vi "Get unpacked Excel file data.vi"(8 "Error In":errorcluster, 10 "temp zip path":path, 11 "Unzipped files":path[](array[path])) -> (0 "Error Out":errorcluster, 1 "workbook.xml path":path, 2 "sheet file names":string[](array[string]), 3 "sheet paths":path[](array[path]), 7 "sharedStrings path":path)   [LabVIEW 2021, in "Files.lvlib"]
uses:
  Files.lvlib
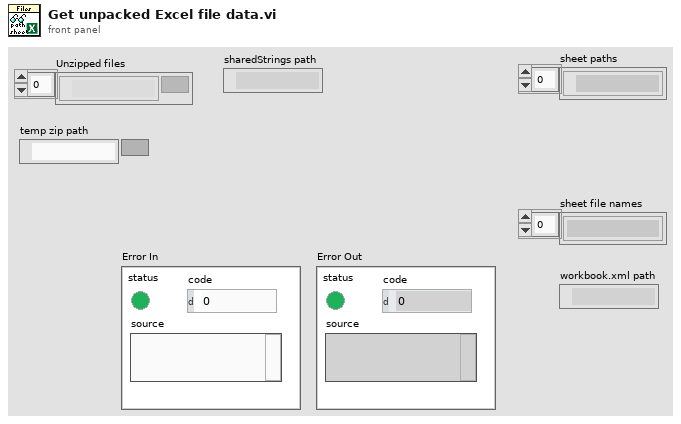
[diagram p1: front panel]
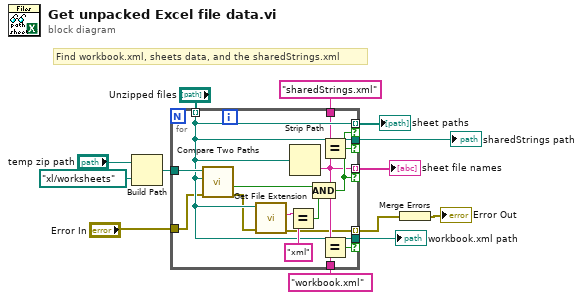
[diagram p0: block diagram]
diagram:
  # "Find workbook.xml, sheets data, and the sharedStrings.xml"
  n1 = Build Path(base path="temp zip path", name or relative path=path "xl/worksheets") -> (appended path=w7:path)
  n2 = for {
    tunnel: "Unzipped files" -> [w23] mode=indexing
    tunnel: [w23] -> w8 if=w26
    tunnel: w7 -> [w28]
    tunnel: [w23] -> w11 mode=indexing if=w21
    tunnel: [w23] -> w9 if=w22
    tunnel: [w20] -> w10 mode=indexing if=w21
    tunnel: "sharedStrings.xml" ("y") -> [w19]
    tunnel: "workbook.xml" ("y") -> [w17]
    tunnel: "Error In" -> [w16]
    tunnel: [w14] -> w2 mode=indexing
    n3 = call <vilib>:"Compare Two Paths.vi"("error in (no error)"=w16, "Path 2"=w23, "Path 1"=w28) -> ("error out"=w15:errorcluster, "Path 2 Relative to Path 1?"=w27:bool)  [unwired: 5 in, 2 out]
    n4 = call <vilib>:"Get File Extension.vi"("error in (no error)"=w15, "file"=w23) -> ("error out"=w14:errorcluster, "lowercase file extension"=w25:string)  [unwired: 5 in, 3 out]
    n5 = Equal?(x=w25, y="xml") -> (x = y?=w18:bool)
    n6 = Strip Path(path=w23) -> (name=w20:string)  [unwired: 1 out]
    n7 = Compound Arithmetic op=AND(w27, w18) -> (w21:bool)
    n8 = Equal?(x=w19, y=w20) -> (x = y?=w26:bool)
    n9 = Equal?(x=w20, y=w17) -> (x = y?=w22:bool)
  }
  "sheet paths" <- w11
  "sheet file names" <- w10
  "workbook.xml path" <- w9
  "sharedStrings path" <- w8
  n10 = Merge Errors(w2) -> (→"Error Out":errorcluster)
